vi "Photodiode.vi"() -> ()   [LabVIEW 2016]
uses:
  controls/ORTForceCurveEnumTypeDef.ctl
  controls/Enum.ctl
  <vilib>/rvi/errors/niLvFpgaAdjustHostInterfaceError.vi
  <vilib>/Utility/error.llb/Error Cluster From Error Code.vi
  controls/FPGAVIreferenceTypeDefScanEngine.ctl
  <vilib>/rvi/interface/nirviReadWriteControl/nirviReadWriteControl.xnode
  FPGA Bitfiles/lbniAFMControlle_scanControl_controllerFPGAPX_N4i+37z1gG8.lvbitx
  NiFpgaLv.dll
panel:
  out "Vert/Horiz":cluster{"Vert":dbl, "Horiz":dbl, "SUM":dbl} {"SUM" format="%_2p"; "Horiz" format="%_2p"; "Vert" format="%_2p"}
  out "Sum":dbl(slide) scale=0.0..10.0 scale format="%-#1_6g"
  out "Photodiode":cluster{"Vert":dbl, "Horiz":dbl, "SUM":dbl}[](graph)
  in  "Range":u16(ring)=1 items=["3V", "10V"]
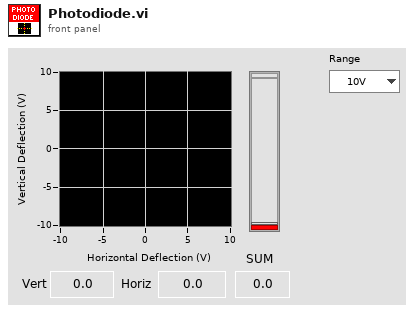
[diagram p1: front panel]
types:
  T1 = typedef "ORTForceCurveEnumTypeDef.ctl" = enum16{"Init", "AskForNewCurve", "Update.CalibZ", "Refresh.Graph", "WaitForEvents", "Close"}
  T2 = typedef "Enum.ctl" = enum16{"Init", "Read", "Write"}
  T3 = typedef "FPGAVIreferenceTypeDefScanEngine.ctl" = refnum<k20>
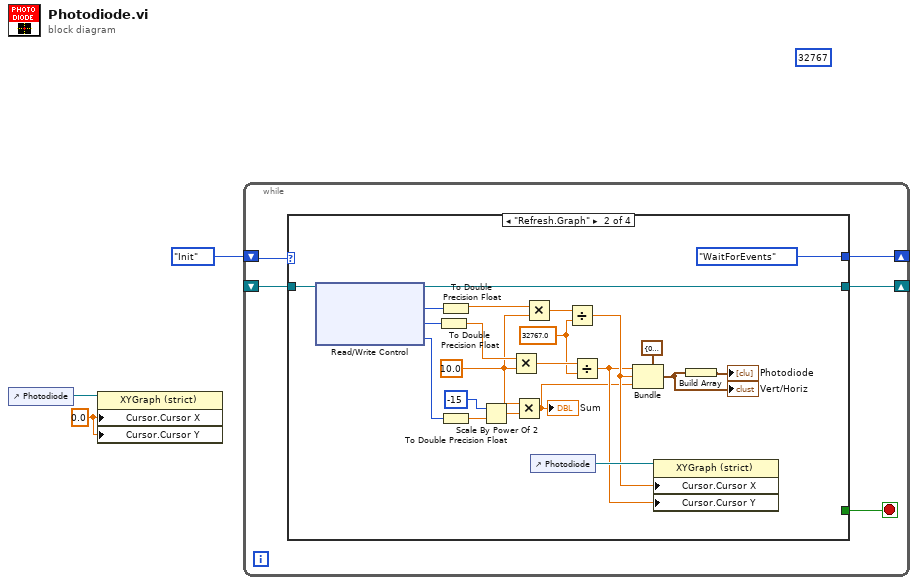
[diagram p0: block diagram]
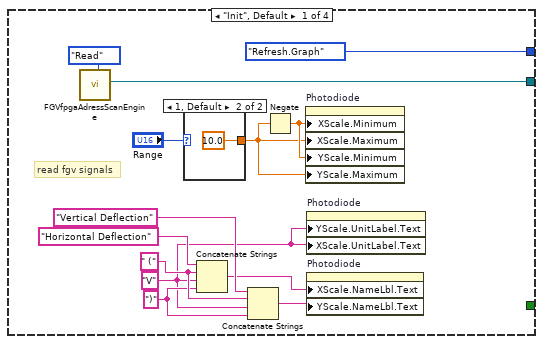
[diagram p2: hidden frame]
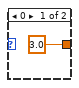
[diagram p3: hidden frame]
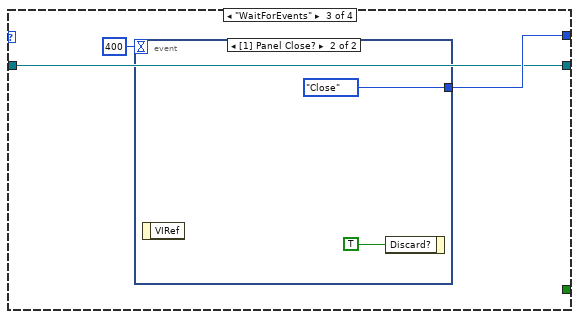
[diagram p4: hidden frame]
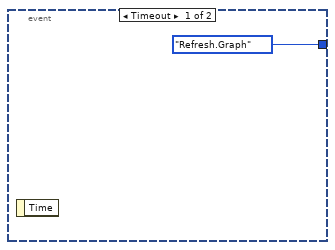
[diagram p5: hidden frame]
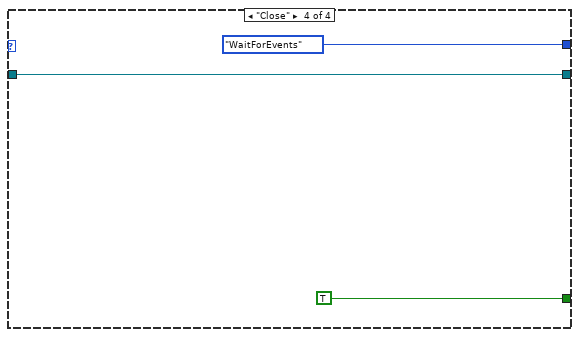
[diagram p6: hidden frame]
diagram:
  (unwired) i16 32767
  w2 = 0.0 ("Cursor.Cursor Position:Cursor X")
  n1 = control-ref of="Photodiode"() -> (w1:refnum<vi>)
  n2 = property class="XYGraph (strict)"(reference=w1, "Cursor.Cursor X"=w2, "Cursor.Cursor Y"=w2) -> ()  [unwired: 1 in, 2 out]
  n3 = while {
    shift-right: [w6] -> _
    shift-left: ORTForceCurveEnumTypeDef."Init" -> [w8]
    shift-right: [w5] -> _
    shift-left: _ -> [w4]
    stop <- w7 stop-if-true
    n4 = case shown="\"Refresh.Graph\"" w8 {
      tunnel: [_ _ _ TRUE] -> w7
      tunnel: [ORTForceCurveEnumTypeDef."Refresh.Graph" ORTForceCurveEnumTypeDef."WaitForEvents" w48 ORTForceCurveEnumTypeDef."WaitForEvents"] -> w6
      tunnel: [w9 w43 w46 w52] -> w5
      tunnel: w4 -> [_ w44 w46 w52]
      frame "Init", Default {
        w15 = " (" ("string")
        w14 = ")" ("string")
        w11 = "V" ("Y Scale.Unit Label.Text")
        # "read fgv signals"
        n5 = call "FGVfpgaAdressScanEngine.vi"("Enum"=Enum."Read") -> ("FPGA.SEout"=w9:T3)  [unwired: 6 in, 4 out]
        n6 = case shown="1, Default" "Range" {
          tunnel: [3.0 10.0] -> w19
          frame 0 {
          }
          frame 1, Default {
          }
        }
        n7 = Concatenate Strings("Horizontal Deflection" ("X Scale.Name Label.Text"), w15, w11, w14) -> (w12:string)
        n8 = Concatenate Strings("Vertical Deflection" ("X Scale.Name Label.Text"), w15, w11, w14) -> (w13:string)
        n9 = Negate(x=w19) -> (-x=w20:dbl)
        n10 = property on="Photodiode" class="XYGraph (strict)"("XScale.Minimum"=w20, "XScale.Maximum"=w19, "YScale.Minimum"=w20, "YScale.Maximum"=w19) -> ()  [unwired: 2 in, 2 out]
        n11 = property on="Photodiode" class="XYGraph (strict)"("YScale.UnitLabel.Text"=w11, "XScale.UnitLabel.Text"=w11) -> ()  [unwired: 2 in, 2 out]
        n12 = property on="Photodiode" class="XYGraph (strict)"("XScale.NameLbl.Text"=w12, "YScale.NameLbl.Text"=w13) -> ()  [unwired: 2 in, 2 out]
      }
      frame "Refresh.Graph" {
        w27 = 10.0 ("y")
        w26 = 32767.0 ("x*y")
        n13 = xnode "Read/Write Control"("FPGA VI Reference In"=w44) -> ("FPGA VI Reference Out"=w43:T3, "aio.s.slowHoriz"=w40:i16, "aio.s.slowVertical"=w39:i16, "aio.s.sum"=w37:i16)  [unwired: 1 in, 1 out]
        n14 = To Double Precision Float(number=w39) -> (double precision float=w33:dbl)
        n15 = To Double Precision Float(number=w40) -> (double precision float=w35:dbl)
        n16 = To Double Precision Float(number=w37) -> (double precision float=w29:dbl)
        n17 = Scale By Power Of 2(n=i16 -15, x=w29) -> (x*2^n=w30:dbl)
        n18 = Multiply(x=w33, y=w27) -> (x*y=w34:dbl)
        n19 = Multiply(x=w27, y=w30) -> (x*y=w24:dbl)
        "Sum" <- w24
        n20 = Multiply(x=w35, y=w27) -> (x*y=w36:dbl)
        n21 = control-ref of="Photodiode"() -> (w42:refnum<vi>)
        n22 = Divide(x=w36, y=w26) -> (x/y=w32:dbl)
        n23 = Divide(x=w34, y=w26) -> (x/y=w31:dbl)
        n24 = Bundle(cluster=cluster{"Vert":dbl, "Horiz":dbl, "SUM":dbl} {"Vert"=0.0, "Horiz"=0.0, "SUM"=0.0} ("Vert/Horiz"), "Vert"=w31, "Horiz"=w32, "SUM"=w24) -> (w38:cluster{"Vert":dbl, "Horiz":dbl, "SUM":dbl})
        "Vert/Horiz" <- w38
        n25 = property class="XYGraph (strict)"(reference=w42, "Cursor.Cursor X"=w32, "Cursor.Cursor Y"=w31) -> ()  [unwired: 1 in, 2 out]
        n26 = Build Array(w38) -> (→"Photodiode":cluster{"Vert":dbl, "Horiz":dbl, "SUM":dbl}[])
      }
      frame "WaitForEvents" {
        n27 = event shown="[1] Panel Close?" {
          selector: _ -> [_ _]
          dyn-events: _ -> [_ _]
          timeout: 400 -> [_ _]
          tunnel: [ORTForceCurveEnumTypeDef."Refresh.Graph" ORTForceCurveEnumTypeDef."Close"] -> w48
          event Timeout {
            n28 = event-data() -> ()  [unwired: 1 in, 1 out]
          }
          event Panel Close? {
            n29 = event-data() -> ()  [unwired: 1 in, 1 out]
            n30 = event-data("Discard?"=TRUE) -> ()  [unwired: 1 in, 1 out]
          }
        }
      }
      frame "Close" {
      }
    }
  }
